vi "Service Request Enable.vi"(0 "VISA resource name":refnum<visa-resource-name>, 5 "Service Request Enable":T1, 11 "error in (no error)":errorcluster) -> (4 "VISA resource name out":refnum<visa-resource-name>, 15 "error out":errorcluster)   [LabVIEW 2012, in "NH Research Regenerative Test Series.lvlib"]
doc: "Service Request enable register controls which bits from the Status Byte should be used to generate a service request when the bit value = 1.\n\nThe Service Request Enable Register consists of the following 8 bits.\n\nBit 0: Module is Busy\nBit 1: Module in Remote Mode\nBit 2: Error in Queue\nBit 3: QUES = Questionable Status Summary\nBit 4: MAV = Message Available\nBit 5: ESB = Event Status Byte Summary\nBit 6: RQS = Request for Service\nBit 7: OPER = Operation Event Summary\n\n\nExample:\n\nIf the user wants to generate SRQ(Service Request) when there is a Message Available and Error in the Queue only, the binary mask 00010100 (0x14) should be used."
uses:
  <instrlib>/NH Research Regenerative Test Series/NH Research Regenerative Test Series.lvlib
panel:
  # "Bit 0: Module is Busy\nBit 1: Module in Remote Mode\nBit 2: Error in Queue\nBit 3: QUES = Questionable Status Summary\nBit 4: MAV = Message Available\nBit 5: ESB = Event Status Byte Summary\nBit 6: RQS = Request for Service\nBit 7: OPER = Operation Event Summary"
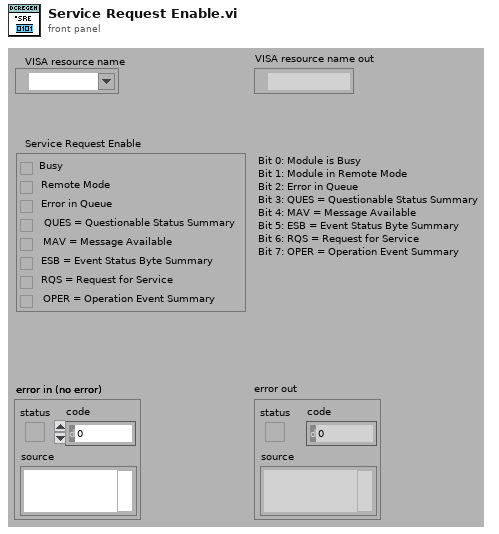
[diagram p1: front panel]
types:
  T1 = cluster{"Busy":bool, "Remote Mode":bool, "Error in Queue":bool, "QUES = Questionable Status Summary":bool, "MAV = Message Available":bool, "ESB = Event Status Byte Summary":bool, "RQS = Request for Service":bool, "OPER = Operation Event Summary":bool}
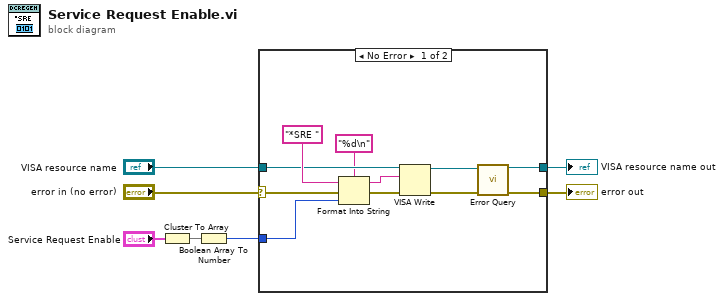
[diagram p0: block diagram]
diagram:
  n1 = Cluster To Array(cluster="Service Request Enable") -> (array=w3:bool[])
  n2 = Boolean Array To Number(Boolean array=w3) -> (number=w1:u32)
  n3 = case shown="No Error" "error in (no error)" {
    selector: "error in (no error)" -> [w14 w19]
    tunnel: w1 -> [w18 _]
    tunnel: "VISA resource name" -> [w13 w20]
    tunnel: [w12 w20] -> w4
    tunnel: [w11 w19] -> w5
    frame No Error {
      n4 = Format Into String(format string="%d\n", initial string="*SRE " ("Command to Send"), error in=w14, w18) -> (resulting string=w16:string, error out=w15:errorcluster)
      n5 = VISA Write(VISA resource name=w13, write buffer=w16, error in (no error)=w15) -> (VISA resource name out=w9:refnum<visa-resource-name>, error out=w8:errorcluster)  [unwired: 1 out]
      n6 = call <instrlib>:"Error Query.vi"("VISA resource name"=w9, "error in (no error)"=w8) -> ("VISA resource name out"=w12:refnum<visa-resource-name>, "error out"=w11:errorcluster)  [unwired: 10 in, 2 out]
    }
    frame Error {
    }
  }
  "error out" <- w5
  "VISA resource name out" <- w4
